vi "Gif.GlobalColorTable.vi"(0 "data":string, 2 "Logical Screen Descriptor":T1, 9 "offset":i32, 11 "error in (no error)":errorcluster) -> (4 "data out":string, 6 "global color table":u32[](array[numeric]), 10 "offset out":i32, 15 "error out":errorcluster)   [LabVIEW 2011]
uses:
  Gif.LogicalScreenDescriptior.ctl
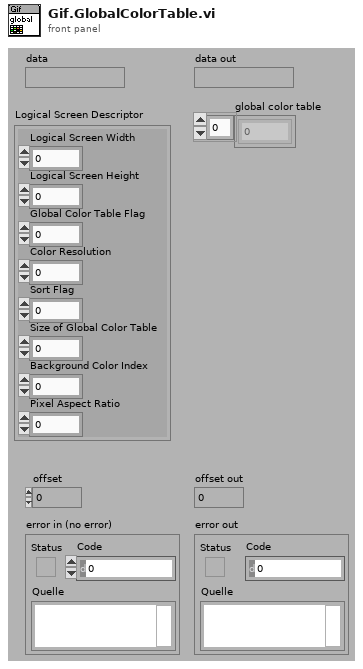
[diagram p1: front panel]
types:
  T1 = typedef "Gif.LogicalScreenDescriptior.ctl" = cluster{"Logical Screen Width":u16, "Logical Screen Height":u16, "Global Color Table Flag":u8, "Color Resolution":u8, "Sort Flag":u8, "Size of Global Color Table":u8, "Background Color Index":u8, "Pixel Aspect Ratio":u8}
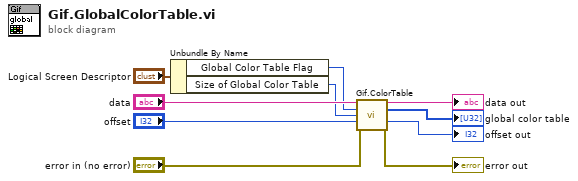
[diagram p0: block diagram]
diagram:
  n1 = Unbundle By Name("Logical Screen Descriptor") -> ("Global Color Table Flag"=w4:u8, "Size of Global Color Table"=w3:u8)
  n2 = call "Gif.ColorTable.vi"("data"="data", "flag"=w4, "Size of Color Table"=w3, "offset"="offset", "error in (no error)"="error in (no error)") -> ("data out"=→"data out":string, "color table"=→"global color table":u32[], "offset out"=→"offset out":i32, "error out"=→"error out":errorcluster)  [unwired: 7 out]
